vi "EdwardsTo_mBar.vi"(1 "Input":string) -> (0 "mBar":dbl)   [LabVIEW 2020]
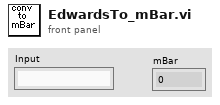
[diagram p1: front panel]
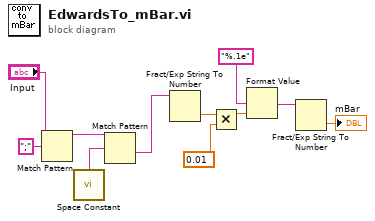
[diagram p0: block diagram]
diagram:
  n1 = Match Pattern(string="Input", regular expression=";") -> (before substring=w10:string)  [unwired: 1 in, 3 out]
  n2 = call <vilib>:"Space Constant.vi"() -> ("String"=w9:string)
  n3 = Match Pattern(string=w10, regular expression=w9) -> (after substring=w5:string)  [unwired: 1 in, 3 out]
  n4 = Fract/Exp String To Number(string=w5) -> (number=w8:dbl)  [unwired: 3 in, 1 out]
  n5 = Multiply(x=w8, y=0.01) -> (x*y=w6:dbl)
  n6 = Format Value(format string="%.1e", value (0)=w6) -> (output string=w3:string)  [unwired: 1 in]
  n7 = Fract/Exp String To Number(string=w3) -> (number=→"mBar":dbl)  [unwired: 3 in, 1 out]
